vi "Create.vi"(8 "error in (no error)":errorcluster, 10 "Desired Stream Specification":T1, 11 "Device ID":string) -> (0 "error out":errorcluster, 3 "Stream":refnum<class "Stream.lvclass">)   [LabVIEW 2020, in "capture.lvlib" / "Stream.lvclass"]
doc: "Create a Stream for the device with the specified parameters. \n\nUse Enumerate Capture Devices.vi to get the Device IDs and Supported Streams."
uses:
  Stream.lvclass
  Stream Specification.ctl
  common/Image Size (Integer).ctl
  Frames per Second.ctl
  Stream.lvclass/Stream.ctl
  common/common.lvlib
  common/bin/gartoolkit_32-1.dll
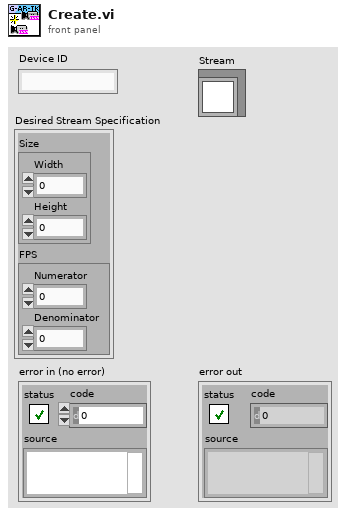
[diagram p1: front panel]
types:
  T1 = typedef "capture.lvlib/Stream.lvclass/Stream Specification.ctl" = cluster{"Size":T2, "FPS":T3}
  T2 = typedef "common.lvlib/Image Size (Integer).ctl" = cluster{"Width":u16, "Height":u16}
  T3 = typedef "capture.lvlib/Stream.lvclass/Frames per Second.ctl" = cluster{"Numerator":u32, "Denominator":u32}
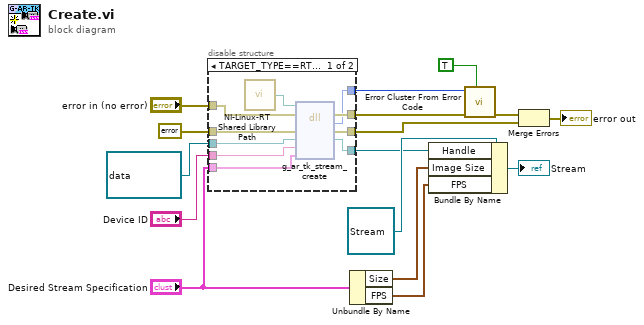
[diagram p0: block diagram]
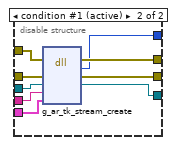
[diagram p2: hidden frame]
diagram:
  n1 = disable-structure shown="TARGET_TYPE==RT&&OS==Linux" {
    disable-tunnel: "error in (no error)" -> [w25 w35]
    disable-tunnel: errorcluster {"status"=FALSE, "code"=0, "source"=""} ("error constant") -> [w24 w34]
    disable-tunnel: refnum<data-value> refnum ("EDVR") -> [w23 w33]
    disable-tunnel: "Device ID" -> [w22 w32]
    disable-tunnel: "Desired Stream Specification" -> [w21 w31]
    disable-tunnel: [w20 w30] -> w5
    disable-tunnel: [w19 w29] -> w4
    disable-tunnel: [w18 w28] -> w3
    disable-tunnel: [w17 w27] -> w2
    frame condition #0 {
      n2 = call "NI-Linux-RT Shared Library Path.vi"() -> ("Path"=w26:path)
      n3 = dll-call lib="?" fn="g_ar_tk_stream_create" ("g_ar_toolkit.*.*:g_ar_tk_capture_stream_create")(path in=w26, error in=w25, "error_cluster"=w24, "EDVR_strm"=w23, "device_id"=w22, "stream_type"=w21) -> (error out=w20:errorcluster, "MgErr"=w19:i32, "error_cluster"=w18:errorcluster, "EDVR_strm"=w17:refnum<data-value>)  [unwired: 3 in, 1 out]
    }
    frame condition #1 (active) {
      n4 = dll-call lib="C:/serenial/lib/g-augmented-reality-toolkit/LabVIEW/common/bin/gartoolkit_*-1.*" fn="g_ar_tk_stream_create" ("g_ar_toolkit.*.*:g_ar_tk_capture_stream_create")(error in=w35, "error_cluster"=w34, "EDVR_strm"=w33, "device_id"=w32, "stream_type"=w31) -> (error out=w30:errorcluster, "MgErr"=w29:i32, "error_cluster"=w28:errorcluster, "EDVR_strm"=w27:refnum<data-value>)  [unwired: 4 in, 1 out]
    }
  }
  n5 = Unbundle By Name("Desired Stream Specification") -> ("Size"=w12:T2, "FPS"=w11:T3)
  n6 = Bundle By Name(cluster=refnum<class "Stream.lvclass"> refnum ("g_ar_toolkit.capture.lvlib:Stream.lvclass"), "Handle"=w2, "Image Size"=w12, "FPS"=w11) -> (→"Stream":refnum<class "Stream.lvclass">)
  n7 = call <vilib>:"Error Cluster From Error Code.vi"("show call chain? (False)"=TRUE, "error in (no error)"=w5, "error code (0)"=w4) -> ("error out"=w16:errorcluster)  [unwired: 6 in]
  n8 = Merge Errors(w16, w3) -> (→"error out":errorcluster)
